vi "HEWH Final Data Check.vi"(4 "Station Message":string="MessageA", 6 "Input State":string="Add Final Data A", 7 "Calc and Calibration in":T3, 8 "error in (no error)":errorcluster, 9 "Reset Cycle Count":bool, 10 "Updated File Path A in":T1, 11 "Log Data Output (A)":bool) -> (0 "error out":errorcluster, 1 "Updated File Path A out":T1, 2 "Calc and Calibration out":T3, 3 "Output State":string)   [LabVIEW 2016]
uses:
  Type Definitions/HEWH Calc and Calibration.ctl
  Utility/Save File/File Setup (Public)/Type Definition/Save File DOE File Path Control.ctl
  Utility/Save File/File Setup (Public)/Type Definition/Save File DOE Data Save Filepaths.ctl
  Utility/Type Definitions/UTILITY Notifier.ctl
  Utility/Save File/File Setup.lvlib
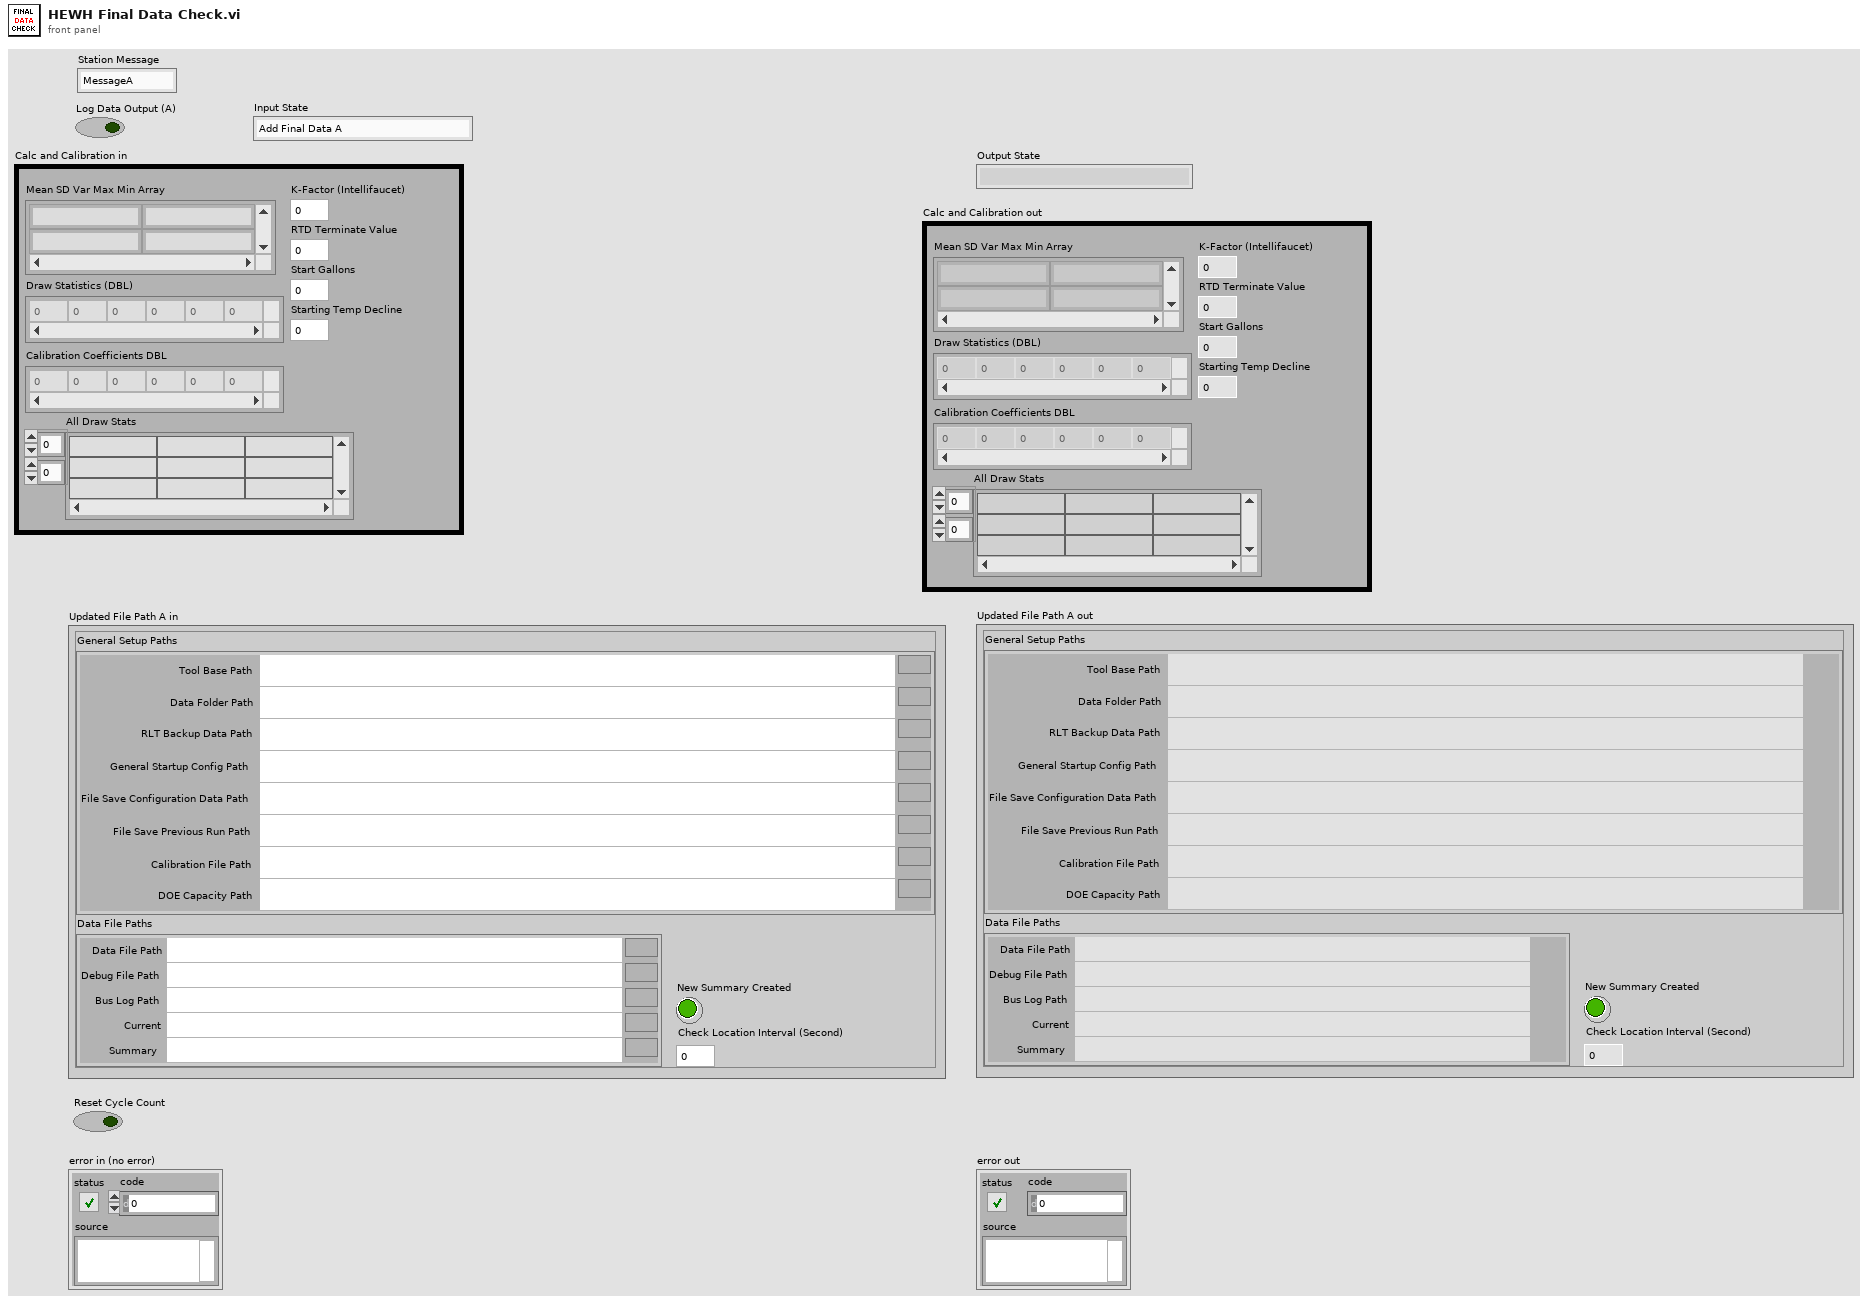
[diagram p1: front panel]
types:
  T1 = typedef "File Setup.lvlib/Save File DOE File Path Control.ctl" = cluster{"General Setup Paths":cluster{"Calibration File Path":path, "DOE Capacity Path":path, "Data Folder Path":path, "RLT Backup Data Path":path, "Tool Base Path":path, "General Startup Config Path":path, "File Save Previous Run Path":path, "File Save Configuration Data Path":path}, "Data File Paths":T2, "New Summary Created":bool, "Check Location Interval (Second)":i32}
  T2 = typedef "File Setup.lvlib/Save File DOE Data Save Filepaths.ctl" = cluster{"Data File Path":path, "Debug File Path":path, "Bus Log Path":path, "Current":path, "Summary":path}
  T3 = typedef "HEWH Calc and Calibration.ctl" = cluster{"Mean SD Var Max Min Array":string[][], "Draw Statistics (DBL)":dbl[][], "Calibration Coefficients DBL":dbl[][], "Start Gallons":dbl, "Starting Temp Decline":dbl, "K-Factor (Intellifaucet)":dbl, "All Draw Stats":string[][], "RTD Terminate Value":dbl}
  T4 = typedef "UTILITY Notifier.ctl" = enum16{"Set", "Read", "Release Ref"}
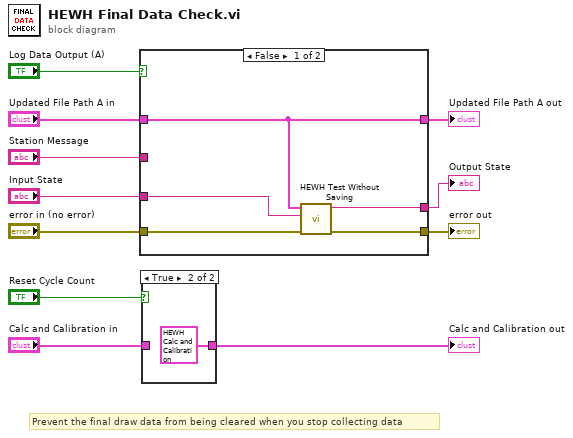
[diagram p0: block diagram]
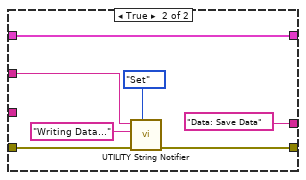
[diagram p3: hidden frame]
diagram:
  # "Prevent the final draw data from being cleared when you stop collecting data"
  n1 = case shown="False" "Log Data Output (A)" {
    tunnel: [w16 "Data: Save Data" ("State(s) in Front (\"\")")] -> w4
    tunnel: "error in (no error)" -> [w15 w20]
    tunnel: [w14 w19] -> w6
    tunnel: "Updated File Path A in" -> [w13 w18]
    tunnel: [w13 w18] -> w8
    tunnel: "Input State" -> [w12 _]
    tunnel: "Station Message" -> [_ w17]
    frame False {
      n2 = call "HEWH Test Without Saving.vi"("Error In"=w15, "State Input"=w12, "Updated File Path C"=w13) -> ("Error Out"=w14:errorcluster, "SM States"=w16:string)  [unwired: 7 in]
    }
    frame True {
      n3 = call "UTILITY String Notifier.vi"("Status"=UTILITY_Notifier."Set", "error in (no error)"=w20, "Set Status"="Writing Data...", "name (unnamed)"=w17) -> ("error out"=w19:errorcluster)  [unwired: 6 in, 1 out]
    }
  }
  "Updated File Path A out" <- w8
  "error out" <- w6
  "Output State" <- w4
  n4 = case shown="True" "Reset Cycle Count" {
    tunnel: "Calc and Calibration in" -> [w24 _]
    tunnel: [w24 T3 {"Mean SD Var Max Min Array"=[], "Draw Statistics (DBL)"=[], "Calibration Coefficients DBL"=[], "Start Gallons"=0.0, "Starting Temp Decline"=1000.0, "K-Factor (Intellifaucet)"=0.0, "All Draw Stats"=[], "RTD Terminate Value"=0.0} ("Calc and Calibration")] -> w10
    frame False {
    }
    frame True {
    }
  }
  "Calc and Calibration out" <- w10
